vi "NewTCPClientDialog.vi"() -> (16 "执行结束":bool)   [LabVIEW 2019]
uses:
  02 Mode/TCPClientMode/TCPClientClass.lvclass
panel:
  in  "取消":bool
  in  "确认":bool
  in  "客服端参数":cluster{"本机端口":u16, "连接方 IP":string, "连接端口":u16}={"本机端口"=5001, "连接方 IP"="127.0.0.1", "连接端口"=4001}
  in  "停止":bool
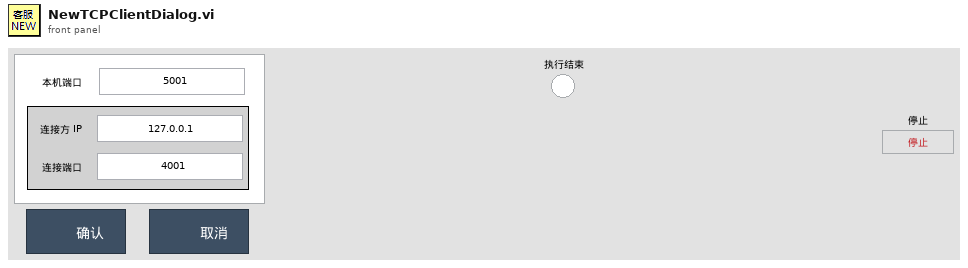
[diagram p1: front panel]
types:
  T1 = map{string, refnum<class "TCPClientClass.lvclass">}
  T2 = cluster{"客服名":string, "客服类":refnum<class "TCPClientClass.lvclass">}
  T3 = cluster{"结果字符串":string, "TCPClientClass 输出":refnum<class "TCPClientClass.lvclass">}
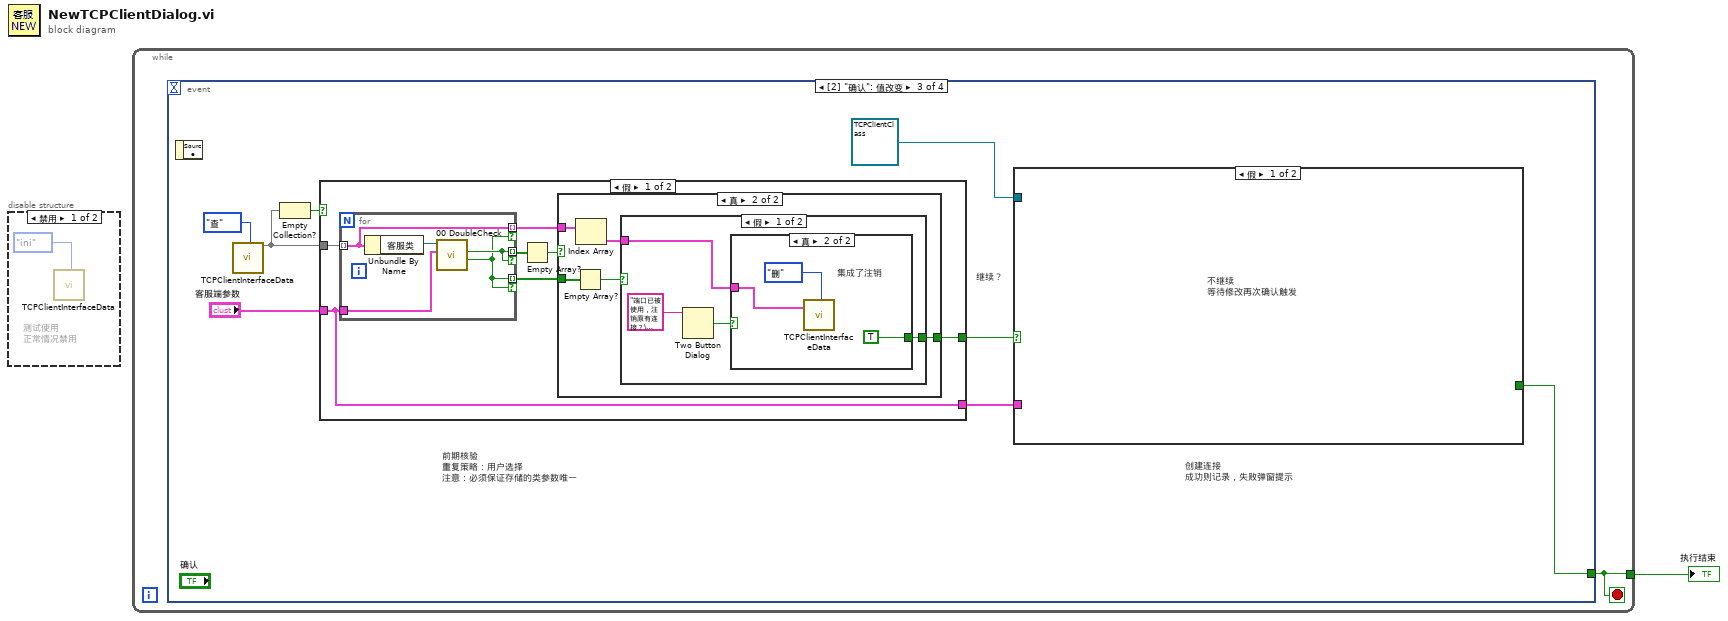
[diagram p0: block diagram]
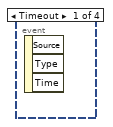
[diagram p3: hidden frame]
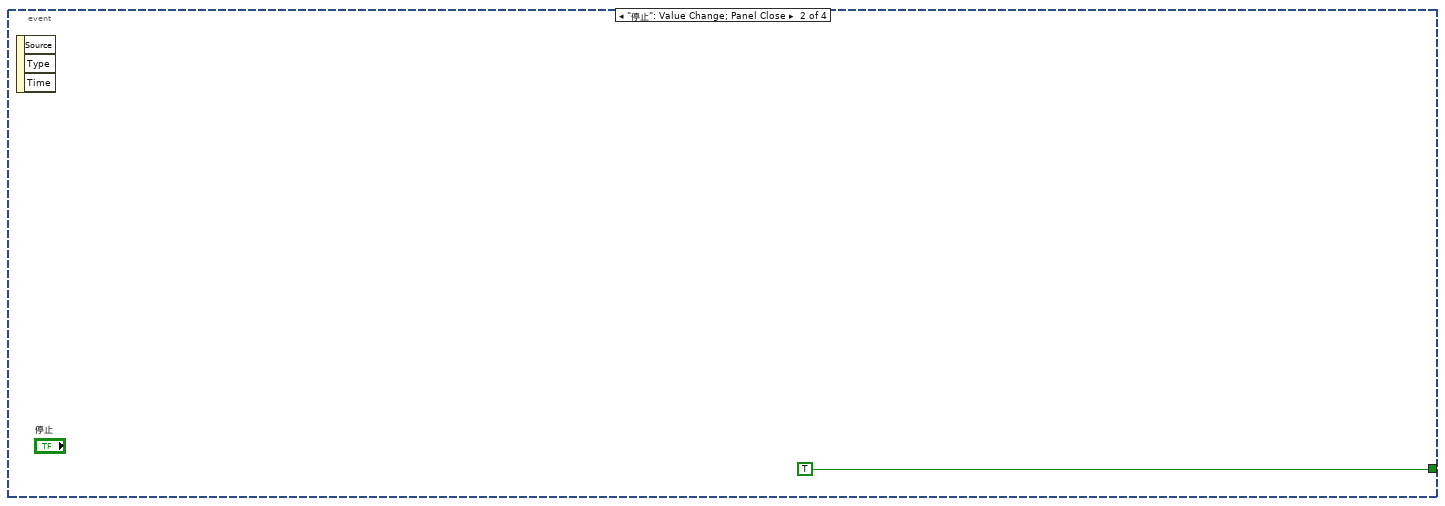
[diagram p4: hidden frame]
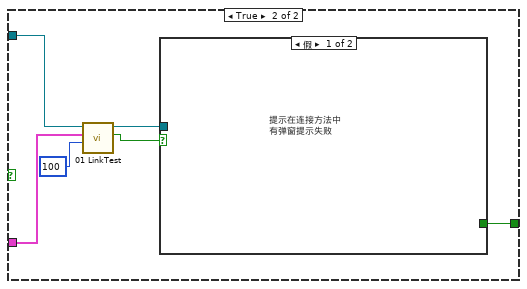
[diagram p5: hidden frame]
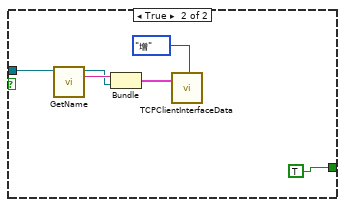
[diagram p6: hidden frame]
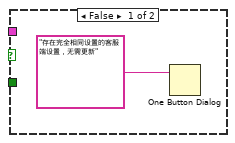
[diagram p7: hidden frame]
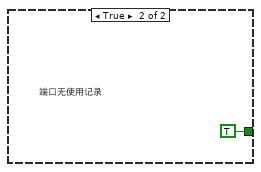
[diagram p9: hidden frame]
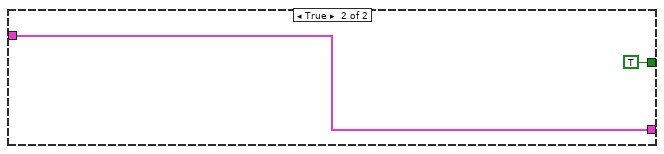
[diagram p10: hidden frame]
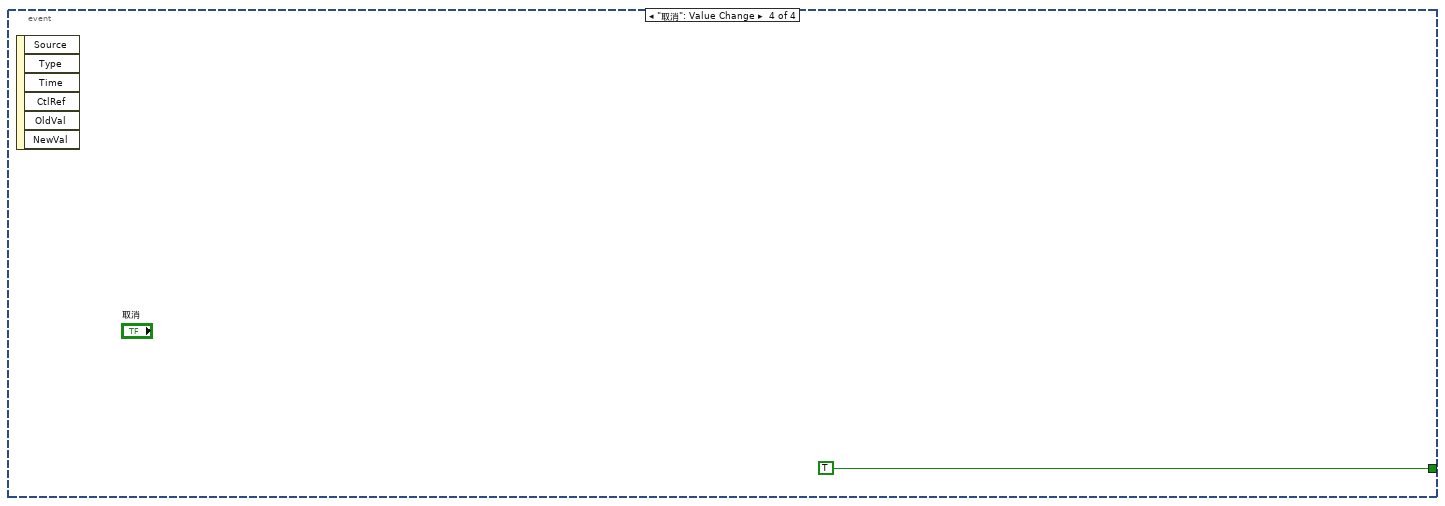
[diagram p11: hidden frame]
diagram:
  n1 = disable-structure shown="禁用" {
    frame Disabled {
      # "测试使用\n正常情况禁用"
      n2 = call "TCPClientInterfaceData.vi"("客服接口枚举"=enum16{"ini", "增", "删", "查", "改"}."ini") -> ()  [unwired: 17 in, 2 out]
    }
    frame Enabled {
    }
  }
  n3 = while {
    tunnel: [w3] -> w1
    stop <- w3 stop-if-true
    n4 = event shown="[2] \"确认\": 值改变" {
      selector: _ -> [_ _ _ _]
      dyn-events: _ -> [_ _ _ _]
      timeout: _ -> [_ _ _ _]
      tunnel: [_ TRUE w5 TRUE] -> w3
      event Timeout {
        n5 = event-data() -> ()  [unwired: 1 in, 3 out]
      }
      event "停止": Value Change; Panel Close {
        n6 = event-data() -> ()  [unwired: 1 in, 3 out]
      }
      event "确认": Value Change {
        # "创建连接\n成功则记录，失败弹窗提示"
        # "继续？"
        # "前期核验\n重复策略：用户选择\n注意：必须保证存储的类参数唯一"
        n7 = event-data() -> ()  [unwired: 1 in, 1 out]
        n8 = call "TCPClientInterfaceData.vi"("客服接口枚举"=enum16{"ini", "增", "删", "查", "改"}."查") -> ("客服表"=w10:T1)  [unwired: 17 in, 1 out]
        n9 = Empty Collection?(1:w10) -> (0:w9:bool)
        n10 = case shown="假" w9 {
          tunnel: w10 -> [w31 _]
          tunnel: "客服端参数" -> [w30 w52]
          tunnel: [w30 w52] -> w7
          tunnel: [w25 TRUE] -> w8
          frame False {
            n11 = for {
              tunnel: w31 -> [w46] mode=indexing
              tunnel: w30 -> [w49]
              tunnel: [w48] -> w29 mode=indexing if=w48
              tunnel: [w47] -> w27 mode=indexing if=w47
              tunnel: [w46] -> w26 mode=indexing if=w47
              n12 = Unbundle By Name(w46) -> ("客服类"=w50:refnum<class "TCPClientClass.lvclass">)
              n13 = call-dynamic "00 DoubleCheck.vi"("客服端参数"=w49, "TCPClientClass 输入"=w50) -> ("端口重复？"=w47:bool, "参数重复？"=w48:bool)  [unwired: 6 in, 2 out]
            }
            n14 = Empty Array?(array=w29) -> (empty?=w28:bool)
            n15 = case shown="真" w28 {
              tunnel: w27 -> [_ w37]
              tunnel: w26 -> [_ w36]
              tunnel: [_ w33] -> w25
              frame False {
                n16 = One Button Dialog(message="存在完全相同设置的客服端设置，无需更新" ("消息")) -> ()  [unwired: 1 in, 1 out]
              }
              frame True {
                n17 = Empty Array?(array=w37) -> (empty?=w35:bool)
                n18 = Index Array(array=w36) -> (element=w34:T2)  [unwired: 1 in]
                n19 = case shown="假" w35 {
                  tunnel: w34 -> [w39 _]
                  tunnel: [w38 TRUE] -> w33
                  frame False {
                    n20 = Two Button Dialog(message="端口已被使用，注销原有连接？\n确认注销，取消或关闭放弃改动" ("消息")) -> (T button?=w40:bool)  [unwired: 2 in]
                    n21 = case shown="真" w40 {
                      tunnel: w39 -> [_ w43]
                      tunnel: [_ TRUE] -> w38
                      frame False {
                      }
                      frame True {
                        # "集成了注销"
                        n22 = call "TCPClientInterfaceData.vi"("信息"=w43, "客服接口枚举"=enum16{"ini", "增", "删", "查", "改"}."删") -> ()  [unwired: 16 in, 2 out]
                      }
                    }
                  }
                  frame True {
                    # "端口无使用记录"
                  }
                }
              }
            }
          }
          frame True {
          }
        }
        n23 = case shown="假" w8 {
          tunnel: w7 -> [_ w17]
          tunnel: refnum<class "TCPClientClass.lvclass"> refnum ("TCPClientClass.lvclass") -> [_ w18]
          tunnel: [_ w13] -> w5
          frame False {
            # "不继续\n等待修改再次确认触发"
          }
          frame True {
            n24 = call-dynamic "01 LinkTest.vi"("超时毫秒"=100, "客服端参数"=w17, "TCPClientClass 输入"=w18) -> ("成功？"=w15:bool, "TCPClientClass 输出"=w14:refnum<class "TCPClientClass.lvclass">)  [unwired: 6 in, 1 out]
            n25 = case shown="假" w15 {
              tunnel: w14 -> [_ w23]
              tunnel: [_ TRUE] -> w13
              frame False {
                # "提示在连接方法中\n有弹窗提示失败"
              }
              frame True {
                n26 = call-dynamic "GetName.vi"("TCPClientClass 输入"=w23) -> ("结果字符串"=w22:string, "TCPClientClass 输出"=w21:refnum<class "TCPClientClass.lvclass">)  [unwired: 8 in, 1 out]
                n27 = Bundle("结果字符串"=w22, "TCPClientClass 输出"=w21) -> (w20:T3)  [unwired: 1 in]
                n28 = call "TCPClientInterfaceData.vi"("信息"=w20, "客服接口枚举"=enum16{"ini", "增", "删", "查", "改"}."增") -> ()  [unwired: 16 in, 2 out]
              }
            }
          }
        }
      }
      event "取消": Value Change {
        n29 = event-data() -> ()  [unwired: 1 in, 6 out]
      }
    }
  }
  "执行结束" <- w1
